vi "init_channel.vi"(8 "error in (no error)":errorcluster, 11 "Thorlabs_OSA300_64 in":refnum<class "OSA300.lvclass">) -> (0 "error out":errorcluster, 3 "Thorlabs_OSA300_64 out":refnum<class "OSA300.lvclass">)   [LabVIEW 2010, in "OSA300.lvclass"]
uses:
  OSA300.lvclass
  _OSAchannel_class/OSAchannel.lvclass
  _misc/Thorlabs_FTS_misc.llb/channelType_spectrum.ctl
  OSA20X_misc.lvlib
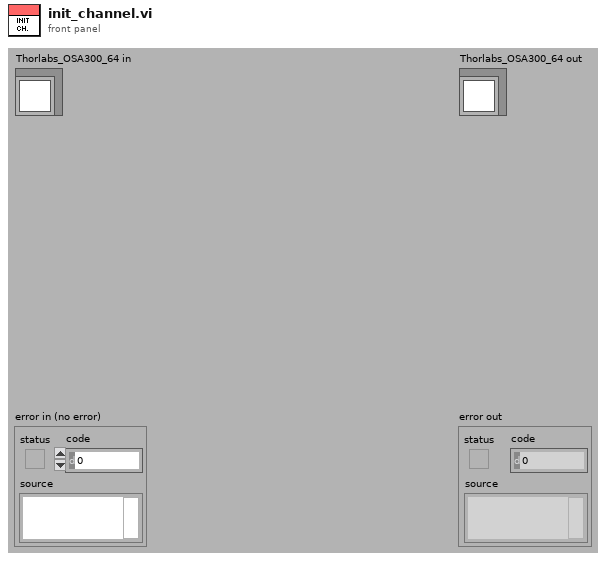
[diagram p1: front panel]
types:
  T1 = typedef "OSA20X_misc.lvlib/channelType_spectrum.ctl" = enum16{"SINGLE CHANNEL", "STICHED"}
  T2 = typedef "OSA300.lvclass/channelType.ctl" = enum16{"REF", "REF_BROADBAND", "DUT1", "DUT2", "DUT3", "DUT4", "unknown"}
  T3 = typedef "OSA20X_misc.lvlib/amplifier_sort.ctl" = enum16{"amp_unknown", "amp_se_8", "amp_se_12_lg", "amp_se_12", "amp_se_16", "amp_diff_8", "amp_diff_12_lg", "amp_diff_12_ir", "amp_diff_16", "amp_other", "amp_other_2"}
  T4 = typedef "OSA20X_misc.lvlib/detector_sort.ctl" = enum16{"unknown", "Silicon", "Silicon PIN", "Silicon MPPC", "InGaAs", "InGaAs ext low", "InGaAs ext high", "InAs", "InAsSb", "InSb", "MCT", "other", "other2", "other3"}
  T5 = typedef "OSA20X_misc.lvlib/interferogram_smoothing.ctl" = enum16{"NONE", "BINOMIAL", "SAVITSKY_GOLAY", "FOURIER", "MOVING_AVERAGE", "GAUSSIAN"}
  T6 = typedef "OSA20X_misc.lvlib/PDTemperatureMode.ctl" = enum16{"cool: better sensitivity/noise floor", "warm: extended wl range"}
  T7 = cluster{"waveMin (cm-1)":sgl, "waveMax (cm-1)":sgl, "gainOffset_auto":bool, "gain":i32, "gain levels nr":u16, "offset":i32, "offset max":u16, "damper available":bool, "damper active":bool, "amplifier sort":T3, "detector sort":T4, "channelIdx global":u16, "spectrIdx":u16, "waveMeter on":bool, "ref gainLevels rel.":refnum<data-value>, "intfgrm_smooth_width":u16, "intfgrm_smooth_nrOfPasses":u16, "intfgrm_smooth":T5, "adc #bits":u16, "temp Variable":bool, "spectr_smooth":T5, "spectr_smooth_width":u16, "spectr_smooth_nrOfPasses":u16, "PD sensitivity mode":T6}
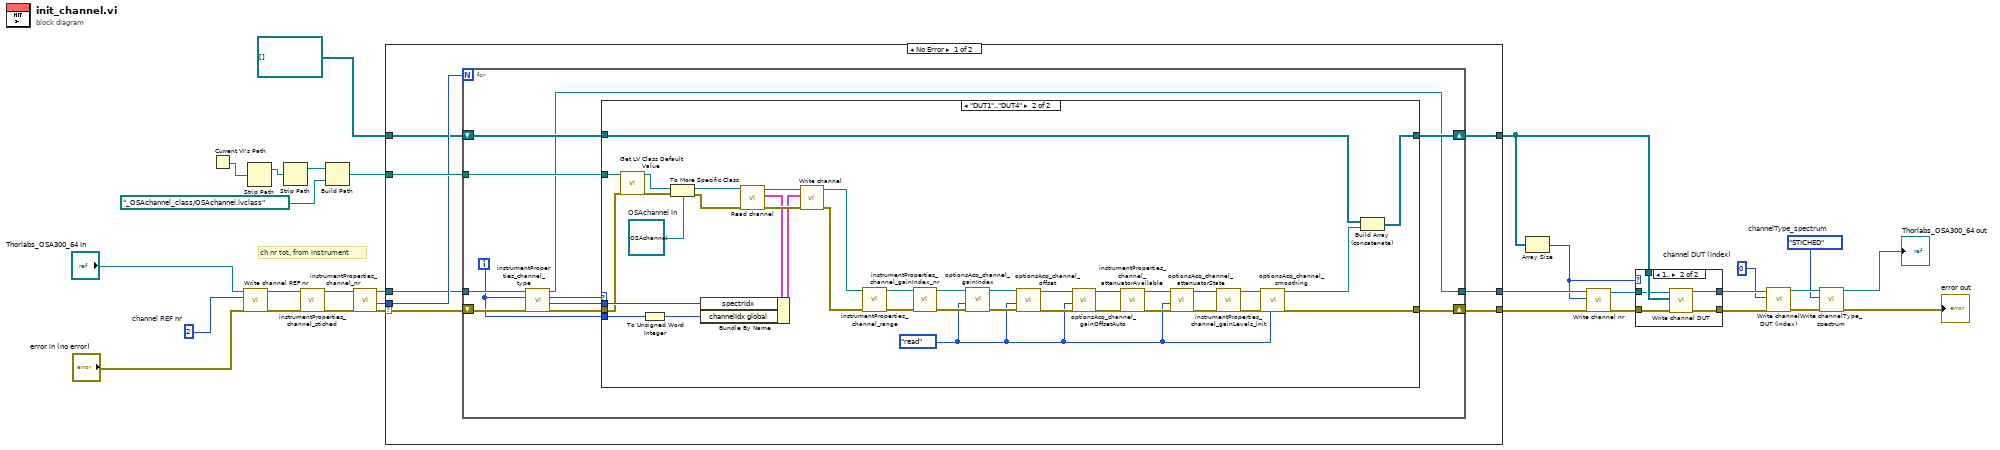
[diagram p0: block diagram]
diagram:
  w1 = channelType_spectrum."STICHED"  # channelType_spectrum
  w12 = 0  # channel DUT (index)
  w22 = 2  # channel REF nr
  # "ch nr tot, from instrument"
  n1 = Current VI's Path() -> (path=w19:path)
  n2 = call "Write channel REF nr.vi"("error in (no error)"="error in (no error)", "channel REF nr"=w22, "OSA300 in"="Thorlabs_OSA300_64 in") -> ("error out"=w27:errorcluster, "OSA300 out"=w26:refnum<class "OSA300.lvclass">)  [unwired: 7 in]
  n3 = Strip Path(path=w19) -> (stripped path=w18:path)  [unwired: 1 out]
  n4 = Strip Path(path=w18) -> (stripped path=w17:path)  [unwired: 1 out]
  n5 = call "instrumentProperties_channel_stiched.vi"("error in (no error)"=w27, "OSA300 in"=w26) -> ("error out"=w24:errorcluster, "OSA300 out"=w25:refnum<class "OSA300.lvclass">)  [unwired: 7 in, 1 out]
  n6 = Build Path(base path=w17, name or relative path=path "_OSAchannel_class/OSAchannel.lvclass") -> (appended path=w16:path)
  n7 = call "instrumentProperties_channel_nr.vi"("error in (no error)"=w24, "OSA300 in"=w25) -> ("error out"=w28:errorcluster, "channels_nr"=w23:i32, "OSA300 out"=w11:refnum<class "OSA300.lvclass">)  [unwired: 7 in]
  n8 = case shown="No Error" w28 {
    selector: w28 -> [w37 w91]
    tunnel: w23 -> [w36 _]
    tunnel: [w34 w91] -> w7
    tunnel: w16 -> [w38 _]
    tunnel: [w33 w90] -> w5
    tunnel: w11 -> [w35 w89]
    tunnel: refnum<class "OSAchannel.lvclass">[] [] -> [w32 w90]
    tunnel: [w31 w89] -> w6
    frame No Error {
      n9 = for {
        N: w36 -> [_]
        tunnel: w38 -> [w49]
        shift-right: [w48] -> w34
        shift-left: w37 -> [w47]
        tunnel: w35 -> [w45]
        shift-right: [w40] -> w33
        shift-left: w32 -> [w41]
        tunnel: [w39] -> w31
        i -> [w43]
        n10 = call "instrumentProperties_channel_type.vi"("error in (no error)"=w47, "channeldx_global"=w43, "OSA300 in"=w45) -> ("error out"=w42:errorcluster, "spectrometerIdx"=w44:u16, "channelType"=w46:T2, "OSA300 out"=w39:refnum<class "OSA300.lvclass">)  [unwired: 5 in]
        n11 = case shown="\"DUT1\"..\"DUT4\"" w46 {
          tunnel: w49 -> [_ w88]
          tunnel: [w51 w52] -> w48
          tunnel: w44 -> [_ w78]
          tunnel: w43 -> [_ w77]
          tunnel: w42 -> [w51 w76]
          tunnel: w41 -> [w50 w61]
          tunnel: [w50 w60] -> w40
          frame "REF", Default {
          }
          frame "DUT1".."DUT4" {
            w54 = enum16{"read", "write"}."read" ("readWrite")
            w85 = refnum<class "OSAchannel.lvclass"> refnum  # OSAchannel in
            n12 = call <vilib>:"Get LV Class Default Value.vi"("error in (no error)"=w76, "class path"=w88) -> ("error out"=w87:errorcluster, "object"=w86:refnum<class>)  [unwired: 8 in]
            n13 = To Unsigned Word Integer(number=w77) -> (unsigned 16bit integer=w57:u16)
            n14 = To More Specific Class(target class=w85, reference=w86, error in=w87) -> (specific class reference=w84:refnum<class "OSAchannel.lvclass">, error out=w83:errorcluster)
            n15 = call "Read channel.vi"("error in (no error)"=w83, "OSAchannel in"=w84) -> ("error out"=w81:errorcluster, "channel"=w80:T7, "OSAchannel out"=w82:refnum<class "OSAchannel.lvclass">)  [unwired: 7 in]
            n16 = Bundle By Name(cluster=w80, "spectrIdx"=w78, "channelIdx global"=w57) -> (w79:T7)
            n17 = call "Write channel.vi"("error in (no error)"=w81, "channel"=w79, "OSAchannel in"=w82) -> ("error out"=w75:errorcluster, "OSAchannel out"=w74:refnum<class "OSAchannel.lvclass">)  [unwired: 7 in]
            n18 = call "instrumentProperties_channel_range.vi"("error in (no error)"=w75, "OSAchannel in"=w74) -> ("error out"=w73:errorcluster, "OSAchannel out"=w72:refnum<class "OSAchannel.lvclass">)  [unwired: 6 in, 2 out]
            n19 = call "instrumentProperties_channel_gainIndex_nr.vi"("error in (no error)"=w73, "OSAchannel in"=w72) -> ("error out"=w67:errorcluster, "OSAchannel out"=w66:refnum<class "OSAchannel.lvclass">)  [unwired: 7 in, 1 out]
            n20 = call "optionsAcq_channel_gainIndex.vi"("error in (no error)"=w67, "readWrite"=w54, "OSAchannel in"=w66) -> ("error out"=w65:errorcluster, "OSAchannel out"=w64:refnum<class "OSAchannel.lvclass">)  [unwired: 5 in, 2 out]
            n21 = call "optionsAcq_channel_offset.vi"("error in (no error)"=w65, "readWrite"=w54, "OSAchannel in"=w64) -> ("error out"=w62:errorcluster, "OSAchannel out"=w63:refnum<class "OSAchannel.lvclass">)  [unwired: 5 in, 2 out]
            n22 = call "optionsAcq_channel_gainOffsetAuto.vi"("error in (no error)"=w62, "readWrite"=w54, "OSAchannel in"=w63) -> ("error out"=w70:errorcluster, "OSAchannel out"=w71:refnum<class "OSAchannel.lvclass">)  [unwired: 5 in, 2 out]
            n23 = call "instrumentProperties_channel_attenuatorAvailable.vi"("error in (no error)"=w70, "OSAchannel in"=w71) -> ("error out"=w69:errorcluster, "OSAchannel out"=w68:refnum<class "OSAchannel.lvclass">)  [unwired: 7 in, 1 out]
            n24 = call "optionsAcq_channel_attenuatorState.vi"("error in (no error)"=w69, "readWrite"=w54, "OSAchannel in"=w68) -> ("error out"=w59:errorcluster, "OSAchannel out"=w58:refnum<class "OSAchannel.lvclass">)  [unwired: 4 in, 3 out]
            n25 = call "instrumentProperties_channel_gainLevels_init.vi"("error in (no error)"=w59, "OSAchannel in"=w58) -> ("error out"=w56:errorcluster, "OSAchannel out"=w55:refnum<class "OSAchannel.lvclass">)  [unwired: 7 in, 1 out]
            n26 = call "optionsAcq_channel_smoothing.vi"("readWrite"=w54, "error in (no error)"=w56, "OSAchannel in"=w55) -> ("error out"=w52:errorcluster, "OSAchannel out"=w53:refnum<class "OSAchannel.lvclass">)  [unwired: 3 in, 4 out]
            n27 = Build Array (concatenate)(w61, w53) -> (w60:refnum<class "OSAchannel.lvclass">[])
          }
        }
      }
    }
    frame Error {
    }
  }
  n28 = Array Size(array=w5) -> (size(s)=w2:i32)
  n29 = call "Write channel nr.vi"("error in (no error)"=w7, "channel nr"=w2, "OSA300 in"=w6) -> ("error out"=w4:errorcluster, "OSA300 out"=w3:refnum<class "OSA300.lvclass">)  [unwired: 7 in]
  n30 = case shown="1.." w2 {
    tunnel: [w92 w98] -> w14
    tunnel: [w93 w97] -> w13
    tunnel: w5 -> [_ w96]
    tunnel: w4 -> [w93 w95]
    tunnel: w3 -> [w92 w94]
    frame 0, Default {
    }
    frame 1.. {
      n31 = call "Write channel DUT.vi"("error in (no error)"=w95, "channel DUT"=w96, "OSA300 in"=w94) -> ("error out"=w97:errorcluster, "OSA300 out"=w98:refnum<class "OSA300.lvclass">)  [unwired: 7 in]
    }
  }
  n32 = call "Write channel DUT (index).vi"("error in (no error)"=w13, "channel DUT (index)"=w12, "OSA300 in"=w14) -> ("error out"=w20:errorcluster, "OSA300 out"=w21:refnum<class "OSA300.lvclass">)  [unwired: 7 in]
  n33 = call "Write channelType_spectrum.vi"("error in (no error)"=w20, "channelType_spectrum"=w1, "OSA300 in"=w21) -> ("error out"=→"error out":errorcluster, "OSA300 out"=→"Thorlabs_OSA300_64 out":refnum<class "OSA300.lvclass">)  [unwired: 7 in]
